vi "Csv_fill_null.vi"(8 "Data in":T1={"Initialisation"={"LMT - Connect UUT (con COM)"="Skip", "LMT - Software Version (rrel)"="Skip", "LMT - Write SKU file (wskuc)"="Skip", "LMT - SKU file name"="Skip", "Connect UUT DDM"="", "Read DDM EOL Timestamp - Mode"="", "Read DDM EOL Timestamp - Timestamp"="", "Read DDM EOL Timestamp - Rig ID"="", "Read DDM EOL Timestamp - Passmark ID"="", "Read DDM EOL Timestamp - Passmark Rev"="", "Software Version before flashing"="", "Read Hardware Serial"="", "UUT DDM SN"="", "Compare DDM SN with MES SN"="Skip", "Backup PCBA Calibration EEPROM Response - CAL"="Skip", "Flash Firmware Version"="", "Check SW Version"="", "Read DDM SW Version after flashing"="", "Set SKU Config"="", "Ready Status"="Skip", "Set Device Mode to EOL"="", "DDM Parameter - Voltage"="", "DDM Parameter - Current"="", "DDM Parameter - Power"="", "DDM Parameter - Speed"="", "DDM Parameter - Pressure"="", "Tester Parameter - Voltage"="", "Tester Parameter - Current"="", "Tester Parameter - Power"="", "Tester Parameter - Ambient Pressure"="", "Tester Parameter - Ambient Temperature"="", "Calculated Parameter - DDM Pressure Corrected"="", "Calculated Parameter - DDM Real Power"="", "Calculated Parameter - Delta V"=""}, "BEMF_Calibration"={"Calibration Result - eol_cold_bemf_temp"="", "DDM Ambient Temp"="Skip", "Restriction Plate Diameter"="Skip", "Calibration Result - eol_bemf_mp_cold_coef_a"="", "Calibration Result - eol_bemf_mp_cold_coef_b"="", "Calibration Result - eol_bemf_mp_cold_coef_c"="", "Calibration Result - eol_bemf_lsi_cold_ref_coeffs"="", "Get - Calibration Result - eol_bemf_lsi_speed"="", "Get - Calibration Result - eol_bemf_lsi_integral_0"="", "Calibration Result - eol_bemf_lsi_integral_1"="", "Get - Calibration Result - eol_bemf_lsi_integral_2"="", "Get - Calibration Result - eol_cold_bemf"="", "Get - Calibration Result - eol_cold_bemf_fisf"="", "Finalise Calibration"="Skip", "Compare -Calibration Result - eol_cold_bemf"="", "Compare -Calibration Result - eol_cold_bemf_fisf"=""}, "ECO"={"Reset Power Tune"="", "Reset BEMF FISF Calibration"="", "Restriction Plate Diameter"="", "ECO - Stabilisation Time"="", "ECO - DDM Parameter - Voltage"="", "ECO - DDM Parameter - Current"="", "ECO - DDM Parameter - Power"="", "ECO - DDM Parameter - Measured Power"="", "ECO - DDM Parameter - Speed"="", "ECO - DDM Parameter - Pressure"="", "ECO - Tester Parameter - Voltage"="", "ECO - Tester Parameter - Current"="", "ECO - Tester Parameter - Power"="", "ECO - Tester Parameter - Ambient Pressure"="", "ECO - Tester Parameter - Ambient Temperature"="", "ECO - Tester Parameter - Ambient Humidity"="", "ECO - Calculated Parameter - DDM Pressure Corrected"="", "ECO - Calculated Parameter - DDM Real Power"="", "ECO - Calculated Parameter - Delta V"="", "ECO - Calculated Parameter - Flowrate"="", "ECO - Calculated Parameter - Airwatt"="", "ECO - Formula"="", "PT ECO - Power Tune Mode Status"="Skip"}, "BOOST"={"Restriction Plate Diameter"="", "BOOST - Stabilisation Time"="", "BOOST - DDM Parameter - Voltage"="", "BOOST - DDM Parameter - Current"="", "BOOST - DDM Parameter - Power"="", "BOOST - DDM Parameter - Measured Power"="", "BOOST - DDM Parameter - Speed"="", "BOOST - DDM Parameter - Pressure"="", "BOOST - Tester Parameter - Voltage"="", "BOOST - Tester Parameter - Current"="", "BOOST - Tester Parameter - Power"="", "BOOST - Tester Parameter - Ambient Pressure"="", "BOOST - Tester Parameter - Ambient Temperature"="", "BOOST - Tester Parameter - Ambient Humidity"="", "BOOST - Calculated Parameter - DDM Pressure Corrected"="", "BOOST - Calculated Parameter - DDM Real Power"="", "BOOST - Calculated Parameter - Delta V"="", "BOOST - Calculated Parameter - Flowrate"="", "BOOST - Calculated Parameter - Airwatt"="", "BOOST - Get AM Presence"="", "Air Muscle Turn Off Status"="", "BOOST - Air Muscle Calculated Parameter - Airwatt B"="", "BOOST - Air Muscle Calculate Airwatt Delta"="", "PT BOOST - Power Tune Mode Status"="Skip", "Finalise Calibration"="Skip", "ECO - Get AW Calibration value"="", "BOOST - Get AW Calibration value"=""}, "MAX"={"Restriction Plate Diameter"="", "MAX - Stabilisation Time"="", "Get Average Delta Tmag (LSIdelta_FISFdelta_LSItmag_FISFtmag_IIRtmag)"="", "Get Average Delta Tmag FISF"="", "MAX - DDM Parameter - Voltage"="", "MAX - DDM Parameter - Current"="", "MAX - DDM Parameter - Power"="", "MAX - DDM Parameter - Measured Power"="", "MAX - DDM Parameter - Speed"="", "MAX - DDM Parameter - Pressure"="", "MAX - Tester Parameter - Voltage"="", "MAX - Tester Parameter - Current"="", "MAX - Tester Parameter - Power"="", "MAX - Tester Parameter - Ambient Pressure"="", "MAX - Tester Parameter - Ambient Temperature"="", "MAX - Tester Parameter - Ambient Humidity"="", "MAX - Calculated Parameter - DDM Pressure Corrected"="", "MAX - Calculated Parameter - DDM Real Power"="", "MAX - Calculated Parameter - Delta V"="", "MAX - Calculated Parameter - Flowrate"="", "MAX - Calculated Parameter - Airwatt"="", "MAX_FISF_Check_Average_Delta_Tmag"="", "MAX - FISF - BEMF Finetune Result"="No BEMF Finetune Required", "MAX tune - Delta P1"="No AW tune required", "MAX tune - Calculated Parameter - Airwatt"="", "Calculate Delta Airwatts - MAX finetune - Delta P2"="No AW finetune required", "MAX finetune - DDM Parameter - Voltage"="", "MAX finetune - DDM Parameter - Current"="", "MAX finetune - DDM Parameter - Power"="", "MAX finetune - DDM Parameter - Measured Power"="", "MAX finetune - DDM Parameter - Speed"="", "MAX finetune - DDM Parameter - Pressure"="", "MAX finetune - Tester Parameter - Voltage"="", "MAX finetune - Tester Parameter - Current"="", "MAX finetune - Tester Parameter - Power"="", "MAX finetune - Tester Parameter - Ambient Pressure"="", "MAX finetune - Tester Parameter - Ambient Temperature"="", "MAX finetune - Tester Parameter - Ambient Humidity"="", "MAX finetune - Calculated Parameter - DDM Pressure Corrected"="", "MAX finetune - Calculated Parameter - DDM Real Power"="", "MAX finetune - Calculated Parameter - Delta V"="", "MAX finetune - Calculated Parameter - Flowrate"="", "MAX finetune - Calculated Parameter - Airwatt"="", "Check Derate Result"="", "Delta Tmag FISF"="", "Get Hot BEMF Result"="", "Calculate delta Pressure"="", "Finalise Calibration"="Skip", "Calculate & Check Delta BEMF"="", "Delta P Airwatts Value"=""}, "LL"={"DDM Ambient Temp"="", "Restriction Plate Diameter"="", "LL - DDM Parameter - Voltage"="", "LL - DDM Parameter - Current"="", "LL - DDM Parameter - Power"="", "LL - DDM Parameter - Measured Power"="", "LL - DDM Parameter - Speed"="", "LL - DDM Parameter - Pressure"="", "LL - Tester Parameter - Voltage"="", "LL - Tester Parameter - Current"="", "LL - Tester Parameter - Power"="", "LL - DDM Real Power"="", "LL - Calibrate Task Detect LL"=""}, "HL"={"HL - DDM Parameter - Voltage"="", "HL - DDM Parameter - Current"="", "HL - DDM Parameter - Power"="", "HL - DDM Parameter - Measured Power"="", "HL - DDM Parameter - Speed"="", "HL - DDM Parameter - Pressure"="", "HL - Tester Parameter - Voltage"="", "HL - Tester Parameter - Current"="", "HL - Tester Parameter - Power"="", "HL - DDM Real Power"="", "HL - Calibrate Task Detect HL"=""}, "LH"={"Restriction Plate Diameter"="", "LH - DDM Parameter - Voltage"="", "LH - DDM Parameter - Current"="", "LH - DDM Parameter - Power"="", "LH - DDM Parameter - Measured Power"="", "LH - DDM Parameter - Speed"="", "LH - DDM Parameter - Pressure"="", "LH - Tester Parameter - Voltage"="", "LH - Tester Parameter - Current"="", "LH - Tester Parameter - Power"="", "LH - DDM Real Power"="", "LH - Calibrate Task Detect LH"=""}, "HH"={"HH - DDM Parameter - Voltage"="", "HH - DDM Parameter - Current"="", "HH - DDM Parameter - Power"="", "HH - DDM Parameter - Measured Power"="", "HH - DDM Parameter - Speed"="", "HH - DDM Parameter - Pressure"="", "HH - Tester Parameter - Voltage"="", "HH - Tester Parameter - Current"="", "HH - Tester Parameter - Power"="", "HH - DDM Real Power"="", "HH - Calibrate Task Detect HH"=""}, "Inlet Blockage Calibration"={"Inlet Blockage Calibration - DDM Parameter - Voltage"="", "Inlet Blockage Calibration - DDM Parameter - Current"="", "Inlet Blockage Calibration - DDM Parameter - Power"="", "Inlet Blockage Calibration - DDM Parameter - Measured Power"="", "Inlet Blockage Calibration - DDM Parameter - Speed"="", "Inlet Blockage Calibration - DDM Parameter - Pressure"="", "Inlet Blockage Calibration - Tester Parameter - Voltage"="", "Inlet Blockage Calibration - Tester Parameter - Current"="", "Inlet Blockage Calibration - Tester Parameter - Power"="", "Inlet Blockage Calibration - DDM Real Power"="", "Calibration Inlet Blockage_E"="", "Finalise Calibration"="Skip", "Get Task Detect LL"="", "Get Task Detect HL"="", "Get Task Detect LH"="", "Get Task Detect HH"="", "Calibration Inlet Blockage"="", "Calibration eol cold bemf temp"=""}, "GOOD"={"GOOD UNIT - Clear EEPROM Error Log"="", "GOOD UNIT - Write Product Timestamp - Mode"="", "GOOD UNIT - Write Product Timestamp - Timestamp"="", "GOOD UNIT - Write Product Timestamp - Rig ID"="", "GOOD UNIT - Write Product Timestamp - Passmark ID"="", "GOOD UNIT - Write Product Timestamp - Passmark Rev"="", "GOOD UNIT - Set Device Mode to PROD"="", "GOOD UNIT - Backup PCBA Calibration EEPROM Response"="", "GOOD UNIT - Check Security Bit"="", "GOOD UNIT - Set Calibration Lock"="", "GOOD UNIT - Get_Calibration_Lock"="", "GOOD UNIT - Disconnect UUT"=""}, "NG"={"NG UNIT - Read NVM Error"="", "NG UNIT - Set Device Mode to FCT"="", "NG UNIT - Backup PCBA Calibration EEPROM Response - CAL"="", "NG UNIT - Backup PCBA Calibration EEPROM Response - ERROR"="", "NG UNIT - Backup PCBA Calibration EEPROM Response - USAGE"="", "NG UNIT - Disconnect UUT"=""}, "SN"="", "Table"=[], "Count"={"Total"=0, "OK"=0, "NG"=0, "Yield"=0.0}, "Start Time"=timestamp(0 s since 1904-01-01), "daemon reference"=refnum, "CT"=0.0, "Config"=[], "OK/NG"=FALSE, "Station ID"="", "MES DDM SN"="Skip", "MES PCBA SN"="", "Retest"="Skip", "Lux"="", "Initialisation_Status"={"LMT - Connect UUT (con COM)"="", "LMT - Software Version (rrel)"="", "LMT - Write SKU file (wskuc)"="", "LMT - SKU file name"="", "Connect UUT DDM"="", "Read DDM EOL Timestamp - Mode"="", "Read DDM EOL Timestamp - Timestamp"="", "Read DDM EOL Timestamp - Rig ID"="", "Read DDM EOL Timestamp - Passmark ID"="", "Read DDM EOL Timestamp - Passmark Rev"="", "Software Version before flashing"="", "Read Hardware Serial"="", "UUT DDM SN"="", "Compare DDM SN with MES SN"="", "Backup PCBA Calibration EEPROM Response - CAL"="", "Flash Firmware Version"="", "Check SW Version"="", "Read DDM SW Version after flashing"="", "Set SKU Config"="", "Ready Status"="", "Set Device Mode to EOL"="", "DDM Parameter - Voltage"="", "DDM Parameter - Current"="", "DDM Parameter - Power"="", "DDM Parameter - Speed"="", "DDM Parameter - Pressure"="", "Tester Parameter - Voltage"="", "Tester Parameter - Current"="", "Tester Parameter - Power"="", "Tester Parameter - Ambient Pressure"="", "Tester Parameter - Ambient Temperature"="", "Calculated Parameter - DDM Pressure Corrected"="", "Calculated Parameter - DDM Real Power"="", "Calculated Parameter - Delta V"=""}, "BEMF_Calibration_Status"={"Calibration Result - eol_cold_bemf_temp"="", "DDM Ambient Temp"="", "Restriction Plate Diameter"="", "Calibration Result - eol_bemf_mp_cold_coef_a"="", "Calibration Result - eol_bemf_mp_cold_coef_b"="", "Calibration Result - eol_bemf_mp_cold_coef_c"="", "Calibration Result - eol_bemf_lsi_cold_ref_coeffs"="", "Get - Calibration Result - eol_bemf_lsi_speed"="", "Get - Calibration Result - eol_bemf_lsi_integral_0"="", "Calibration Result - eol_bemf_lsi_integral_1"="", "Get - Calibration Result - eol_bemf_lsi_integral_2"="", "Get - Calibration Result - eol_cold_bemf"="", "Get - Calibration Result - eol_cold_bemf_fisf"="", "Finalise Calibration"="", "Compare -Calibration Result - eol_cold_bemf"="", "Compare -Calibration Result - eol_cold_bemf_fisf"=""}, "ECO_Status"={"Reset Power Tune"="", "Reset BEMF FISF Calibration"="", "Restriction Plate Diameter"="", "ECO - Stabilisation Time"="", "ECO - DDM Parameter - Voltage"="", "ECO - DDM Parameter - Current"="", "ECO - DDM Parameter - Power"="", "ECO - DDM Parameter - Measured Power"="", "ECO - DDM Parameter - Speed"="", "ECO - DDM Parameter - Pressure"="", "ECO - Tester Parameter - Voltage"="", "ECO - Tester Parameter - Current"="", "ECO - Tester Parameter - Power"="", "ECO - Tester Parameter - Ambient Pressure"="", "ECO - Tester Parameter - Ambient Temperature"="", "ECO - Tester Parameter - Ambient Humidity"="", "ECO - Calculated Parameter - DDM Pressure Corrected"="", "ECO - Calculated Parameter - DDM Real Power"="", "ECO - Calculated Parameter - Delta V"="", "ECO - Calculated Parameter - Flowrate"="", "ECO - Calculated Parameter - Airwatt"="", "ECO - Formula"="", "PT ECO - Power Tune Mode Status"=""}, "BOOST_Status"={"Restriction Plate Diameter"="", "BOOST - Stabilisation Time"="", "BOOST - DDM Parameter - Voltage"="", "BOOST - DDM Parameter - Current"="", "BOOST - DDM Parameter - Power"="", "BOOST - DDM Parameter - Measured Power"="", "BOOST - DDM Parameter - Speed"="", "BOOST - DDM Parameter - Pressure"="", "BOOST - Tester Parameter - Voltage"="", "BOOST - Tester Parameter - Current"="", "BOOST - Tester Parameter - Power"="", "BOOST - Tester Parameter - Ambient Pressure"="", "BOOST - Tester Parameter - Ambient Temperature"="", "BOOST - Tester Parameter - Ambient Humidity"="", "BOOST - Calculated Parameter - DDM Pressure Corrected"="", "BOOST - Calculated Parameter - DDM Real Power"="", "BOOST - Calculated Parameter - Delta V"="", "BOOST - Calculated Parameter - Flowrate"="", "BOOST - Calculated Parameter - Airwatt"="", "BOOST - Get AM Presence"="", "Air Muscle Turn Off Status"="", "BOOST - Air Muscle Calculated Parameter - Airwatt B"="", "BOOST - Air Muscle Calculate Airwatt Delta"="", "PT BOOST - Power Tune Mode Status"="", "Finalise Calibration"="", "ECO - Get AW Calibration value"="", "BOOST - Get AW Calibration value"=""}, "MAX_Status"={"Restriction Plate Diameter"="", "MAX - Stabilisation Time"="", "Get Average Delta Tmag (LSIdelta_FISFdelta_LSItmag_FISFtmag_IIRtmag)"="", "Get Average Delta Tmag FISF"="", "MAX - DDM Parameter - Voltage"="", "MAX - DDM Parameter - Current"="", "MAX - DDM Parameter - Power"="", "MAX - DDM Parameter - Measured Power"="", "MAX - DDM Parameter - Speed"="", "MAX - DDM Parameter - Pressure"="", "MAX - Tester Parameter - Voltage"="", "MAX - Tester Parameter - Current"="", "MAX - Tester Parameter - Power"="", "MAX - Tester Parameter - Ambient Pressure"="", "MAX - Tester Parameter - Ambient Temperature"="", "MAX - Tester Parameter - Ambient Humidity"="", "MAX - Calculated Parameter - DDM Pressure Corrected"="", "MAX - Calculated Parameter - DDM Real Power"="", "MAX - Calculated Parameter - Delta V"="", "MAX - Calculated Parameter - Flowrate"="", "MAX - Calculated Parameter - Airwatt"="", "MAX_FISF_Check_Average_Delta_Tmag"="", "MAX - FISF - BEMF Finetune Result"="", "MAX tune - Delta P1"="", "MAX tune - Calculated Parameter - Airwatt"="", "Calculate Delta Airwatts - MAX finetune - Delta P2"="", "MAX finetune - DDM Parameter - Voltage"="", "MAX finetune - DDM Parameter - Current"="", "MAX finetune - DDM Parameter - Power"="", "MAX finetune - DDM Parameter - Measured Power"="", "MAX finetune - DDM Parameter - Speed"="", "MAX finetune - DDM Parameter - Pressure"="", "MAX finetune - Tester Parameter - Voltage"="", "MAX finetune - Tester Parameter - Current"="", "MAX finetune - Tester Parameter - Power"="", "MAX finetune - Tester Parameter - Ambient Pressure"="", "MAX finetune - Tester Parameter - Ambient Temperature"="", "MAX finetune - Tester Parameter - Ambient Humidity"="", "MAX finetune - Calculated Parameter - DDM Pressure Corrected"="", "MAX finetune - Calculated Parameter - DDM Real Power"="", "MAX finetune - Calculated Parameter - Delta V"="", "MAX finetune - Calculated Parameter - Flowrate"="", "MAX finetune - Calculated Parameter - Airwatt"="", "Check Derate Result"="", "Delta Tmag FISF"="", "Get Hot BEMF Result"="", "Calculate delta Pressure"="", "Finalise Calibration"="", "Calculate & Check Delta BEMF"="", "Delta P Airwatts Value"=""}, "LL_Status"={"DDM Ambient Temp"="", "Restriction Plate Diameter"="", "LL - DDM Parameter - Voltage"="", "LL - DDM Parameter - Current"="", "LL - DDM Parameter - Power"="", "LL - DDM Parameter - Measured Power"="", "LL - DDM Parameter - Speed"="", "LL - DDM Parameter - Pressure"="", "LL - Tester Parameter - Voltage"="", "LL - Tester Parameter - Current"="", "LL - Tester Parameter - Power"="", "LL - DDM Real Power"="", "LL - Calibrate Task Detect LL"=""}, "HL_Status"={"HL - DDM Parameter - Voltage"="", "HL - DDM Parameter - Current"="", "HL - DDM Parameter - Power"="", "HL - DDM Parameter - Measured Power"="", "HL - DDM Parameter - Speed"="", "HL - DDM Parameter - Pressure"="", "HL - Tester Parameter - Voltage"="", "HL - Tester Parameter - Current"="", "HL - Tester Parameter - Power"="", "HL - DDM Real Power"="", "HL - Calibrate Task Detect HL"=""}, "LH_Status"={"Restriction Plate Diameter"="", "LH - DDM Parameter - Voltage"="", "LH - DDM Parameter - Current"="", "LH - DDM Parameter - Power"="", "LH - DDM Parameter - Measured Power"="", "LH - DDM Parameter - Speed"="", "LH - DDM Parameter - Pressure"="", "LH - Tester Parameter - Voltage"="", "LH - Tester Parameter - Current"="", "LH - Tester Parameter - Power"="", "LH - DDM Real Power"="", "LH - Calibrate Task Detect LH"=""}, "HH_Status"={"HH - DDM Parameter - Voltage"="", "HH - DDM Parameter - Current"="", "HH - DDM Parameter - Power"="", "HH - DDM Parameter - Measured Power"="", "HH - DDM Parameter - Speed"="", "HH - DDM Parameter - Pressure"="", "HH - Tester Parameter - Voltage"="", "HH - Tester Parameter - Current"="", "HH - Tester Parameter - Power"="", "HH - DDM Real Power"="", "HH - Calibrate Task Detect HH"=""}, "Inlet Blockage Calibration_Status"={"Inlet Blockage Calibration - DDM Parameter - Voltage"="", "Inlet Blockage Calibration - DDM Parameter - Current"="", "Inlet Blockage Calibration - DDM Parameter - Power"="", "Inlet Blockage Calibration - DDM Parameter - Measured Power"="", "Inlet Blockage Calibration - DDM Parameter - Speed"="", "Inlet Blockage Calibration - DDM Parameter - Pressure"="", "Inlet Blockage Calibration - Tester Parameter - Voltage"="", "Inlet Blockage Calibration - Tester Parameter - Current"="", "Inlet Blockage Calibration - Tester Parameter - Power"="", "Inlet Blockage Calibration - DDM Real Power"="", "Calibration Inlet Blockage_E"="", "Finalise Calibration"="", "Get Task Detect LL"="", "Get Task Detect HL"="", "Get Task Detect LH"="", "Get Task Detect HH"="", "Calibration Inlet Blockage"="", "Calibration eol cold bemf temp"=""}, "GOOD_Status"={"GOOD UNIT - Clear EEPROM Error Log"="", "GOOD UNIT - Write Product Timestamp - Mode"="", "GOOD UNIT - Write Product Timestamp - Timestamp"="", "GOOD UNIT - Write Product Timestamp - Rig ID"="", "GOOD UNIT - Write Product Timestamp - Passmark ID"="", "GOOD UNIT - Write Product Timestamp - Passmark Rev"="", "GOOD UNIT - Set Device Mode to PROD"="", "GOOD UNIT - Backup PCBA Calibration EEPROM Response"="", "GOOD UNIT - Check Security Bit"="", "GOOD UNIT - Set Calibration Lock"="", "GOOD UNIT - Get_Calibration_Lock"="", "GOOD UNIT - Disconnect UUT"=""}, "NG_Status"={"NG UNIT - Read NVM Error"="", "NG UNIT - Set Device Mode to FCT"="", "NG UNIT - Backup PCBA Calibration EEPROM Response - CAL"="", "NG UNIT - Backup PCBA Calibration EEPROM Response - ERROR"="", "NG UNIT - Backup PCBA Calibration EEPROM Response - USAGE"="", "NG UNIT - Disconnect UUT"=""}, "SKU"="", "Plate_Diameter"="", "Alarm"=""}) -> (0 "Data out":T1={"Initialisation"={"LMT - Connect UUT (con COM)"="Skip", "LMT - Software Version (rrel)"="Skip", "LMT - Write SKU file (wskuc)"="Skip", "LMT - SKU file name"="Skip", "Connect UUT DDM"="", "Read DDM EOL Timestamp - Mode"="", "Read DDM EOL Timestamp - Timestamp"="", "Read DDM EOL Timestamp - Rig ID"="", "Read DDM EOL Timestamp - Passmark ID"="", "Read DDM EOL Timestamp - Passmark Rev"="", "Software Version before flashing"="", "Read Hardware Serial"="", "UUT DDM SN"="", "Compare DDM SN with MES SN"="Skip", "Backup PCBA Calibration EEPROM Response - CAL"="Skip", "Flash Firmware Version"="", "Check SW Version"="", "Read DDM SW Version after flashing"="", "Set SKU Config"="", "Ready Status"="Skip", "Set Device Mode to EOL"="", "DDM Parameter - Voltage"="", "DDM Parameter - Current"="", "DDM Parameter - Power"="", "DDM Parameter - Speed"="", "DDM Parameter - Pressure"="", "Tester Parameter - Voltage"="", "Tester Parameter - Current"="", "Tester Parameter - Power"="", "Tester Parameter - Ambient Pressure"="", "Tester Parameter - Ambient Temperature"="", "Calculated Parameter - DDM Pressure Corrected"="", "Calculated Parameter - DDM Real Power"="", "Calculated Parameter - Delta V"=""}, "BEMF_Calibration"={"Calibration Result - eol_cold_bemf_temp"="", "DDM Ambient Temp"="Skip", "Restriction Plate Diameter"="Skip", "Calibration Result - eol_bemf_mp_cold_coef_a"="", "Calibration Result - eol_bemf_mp_cold_coef_b"="", "Calibration Result - eol_bemf_mp_cold_coef_c"="", "Calibration Result - eol_bemf_lsi_cold_ref_coeffs"="", "Get - Calibration Result - eol_bemf_lsi_speed"="", "Get - Calibration Result - eol_bemf_lsi_integral_0"="", "Calibration Result - eol_bemf_lsi_integral_1"="", "Get - Calibration Result - eol_bemf_lsi_integral_2"="", "Get - Calibration Result - eol_cold_bemf"="", "Get - Calibration Result - eol_cold_bemf_fisf"="", "Finalise Calibration"="Skip", "Compare -Calibration Result - eol_cold_bemf"="", "Compare -Calibration Result - eol_cold_bemf_fisf"=""}, "ECO"={"Reset Power Tune"="", "Reset BEMF FISF Calibration"="", "Restriction Plate Diameter"="", "ECO - Stabilisation Time"="", "ECO - DDM Parameter - Voltage"="", "ECO - DDM Parameter - Current"="", "ECO - DDM Parameter - Power"="", "ECO - DDM Parameter - Measured Power"="", "ECO - DDM Parameter - Speed"="", "ECO - DDM Parameter - Pressure"="", "ECO - Tester Parameter - Voltage"="", "ECO - Tester Parameter - Current"="", "ECO - Tester Parameter - Power"="", "ECO - Tester Parameter - Ambient Pressure"="", "ECO - Tester Parameter - Ambient Temperature"="", "ECO - Tester Parameter - Ambient Humidity"="", "ECO - Calculated Parameter - DDM Pressure Corrected"="", "ECO - Calculated Parameter - DDM Real Power"="", "ECO - Calculated Parameter - Delta V"="", "ECO - Calculated Parameter - Flowrate"="", "ECO - Calculated Parameter - Airwatt"="", "ECO - Formula"="", "PT ECO - Power Tune Mode Status"="Skip"}, "BOOST"={"Restriction Plate Diameter"="", "BOOST - Stabilisation Time"="", "BOOST - DDM Parameter - Voltage"="", "BOOST - DDM Parameter - Current"="", "BOOST - DDM Parameter - Power"="", "BOOST - DDM Parameter - Measured Power"="", "BOOST - DDM Parameter - Speed"="", "BOOST - DDM Parameter - Pressure"="", "BOOST - Tester Parameter - Voltage"="", "BOOST - Tester Parameter - Current"="", "BOOST - Tester Parameter - Power"="", "BOOST - Tester Parameter - Ambient Pressure"="", "BOOST - Tester Parameter - Ambient Temperature"="", "BOOST - Tester Parameter - Ambient Humidity"="", "BOOST - Calculated Parameter - DDM Pressure Corrected"="", "BOOST - Calculated Parameter - DDM Real Power"="", "BOOST - Calculated Parameter - Delta V"="", "BOOST - Calculated Parameter - Flowrate"="", "BOOST - Calculated Parameter - Airwatt"="", "BOOST - Get AM Presence"="", "Air Muscle Turn Off Status"="", "BOOST - Air Muscle Calculated Parameter - Airwatt B"="", "BOOST - Air Muscle Calculate Airwatt Delta"="", "PT BOOST - Power Tune Mode Status"="Skip", "Finalise Calibration"="Skip", "ECO - Get AW Calibration value"="", "BOOST - Get AW Calibration value"=""}, "MAX"={"Restriction Plate Diameter"="", "MAX - Stabilisation Time"="", "Get Average Delta Tmag (LSIdelta_FISFdelta_LSItmag_FISFtmag_IIRtmag)"="", "Get Average Delta Tmag FISF"="", "MAX - DDM Parameter - Voltage"="", "MAX - DDM Parameter - Current"="", "MAX - DDM Parameter - Power"="", "MAX - DDM Parameter - Measured Power"="", "MAX - DDM Parameter - Speed"="", "MAX - DDM Parameter - Pressure"="", "MAX - Tester Parameter - Voltage"="", "MAX - Tester Parameter - Current"="", "MAX - Tester Parameter - Power"="", "MAX - Tester Parameter - Ambient Pressure"="", "MAX - Tester Parameter - Ambient Temperature"="", "MAX - Tester Parameter - Ambient Humidity"="", "MAX - Calculated Parameter - DDM Pressure Corrected"="", "MAX - Calculated Parameter - DDM Real Power"="", "MAX - Calculated Parameter - Delta V"="", "MAX - Calculated Parameter - Flowrate"="", "MAX - Calculated Parameter - Airwatt"="", "MAX_FISF_Check_Average_Delta_Tmag"="", "MAX - FISF - BEMF Finetune Result"="No BEMF Finetune Required", "MAX tune - Delta P1"="No AW tune required", "MAX tune - Calculated Parameter - Airwatt"="", "Calculate Delta Airwatts - MAX finetune - Delta P2"="No AW finetune required", "MAX finetune - DDM Parameter - Voltage"="", "MAX finetune - DDM Parameter - Current"="", "MAX finetune - DDM Parameter - Power"="", "MAX finetune - DDM Parameter - Measured Power"="", "MAX finetune - DDM Parameter - Speed"="", "MAX finetune - DDM Parameter - Pressure"="", "MAX finetune - Tester Parameter - Voltage"="", "MAX finetune - Tester Parameter - Current"="", "MAX finetune - Tester Parameter - Power"="", "MAX finetune - Tester Parameter - Ambient Pressure"="", "MAX finetune - Tester Parameter - Ambient Temperature"="", "MAX finetune - Tester Parameter - Ambient Humidity"="", "MAX finetune - Calculated Parameter - DDM Pressure Corrected"="", "MAX finetune - Calculated Parameter - DDM Real Power"="", "MAX finetune - Calculated Parameter - Delta V"="", "MAX finetune - Calculated Parameter - Flowrate"="", "MAX finetune - Calculated Parameter - Airwatt"="", "Check Derate Result"="", "Delta Tmag FISF"="", "Get Hot BEMF Result"="", "Calculate delta Pressure"="", "Finalise Calibration"="Skip", "Calculate & Check Delta BEMF"="", "Delta P Airwatts Value"=""}, "LL"={"DDM Ambient Temp"="", "Restriction Plate Diameter"="", "LL - DDM Parameter - Voltage"="", "LL - DDM Parameter - Current"="", "LL - DDM Parameter - Power"="", "LL - DDM Parameter - Measured Power"="", "LL - DDM Parameter - Speed"="", "LL - DDM Parameter - Pressure"="", "LL - Tester Parameter - Voltage"="", "LL - Tester Parameter - Current"="", "LL - Tester Parameter - Power"="", "LL - DDM Real Power"="", "LL - Calibrate Task Detect LL"=""}, "HL"={"HL - DDM Parameter - Voltage"="", "HL - DDM Parameter - Current"="", "HL - DDM Parameter - Power"="", "HL - DDM Parameter - Measured Power"="", "HL - DDM Parameter - Speed"="", "HL - DDM Parameter - Pressure"="", "HL - Tester Parameter - Voltage"="", "HL - Tester Parameter - Current"="", "HL - Tester Parameter - Power"="", "HL - DDM Real Power"="", "HL - Calibrate Task Detect HL"=""}, "LH"={"Restriction Plate Diameter"="", "LH - DDM Parameter - Voltage"="", "LH - DDM Parameter - Current"="", "LH - DDM Parameter - Power"="", "LH - DDM Parameter - Measured Power"="", "LH - DDM Parameter - Speed"="", "LH - DDM Parameter - Pressure"="", "LH - Tester Parameter - Voltage"="", "LH - Tester Parameter - Current"="", "LH - Tester Parameter - Power"="", "LH - DDM Real Power"="", "LH - Calibrate Task Detect LH"=""}, "HH"={"HH - DDM Parameter - Voltage"="", "HH - DDM Parameter - Current"="", "HH - DDM Parameter - Power"="", "HH - DDM Parameter - Measured Power"="", "HH - DDM Parameter - Speed"="", "HH - DDM Parameter - Pressure"="", "HH - Tester Parameter - Voltage"="", "HH - Tester Parameter - Current"="", "HH - Tester Parameter - Power"="", "HH - DDM Real Power"="", "HH - Calibrate Task Detect HH"=""}, "Inlet Blockage Calibration"={"Inlet Blockage Calibration - DDM Parameter - Voltage"="", "Inlet Blockage Calibration - DDM Parameter - Current"="", "Inlet Blockage Calibration - DDM Parameter - Power"="", "Inlet Blockage Calibration - DDM Parameter - Measured Power"="", "Inlet Blockage Calibration - DDM Parameter - Speed"="", "Inlet Blockage Calibration - DDM Parameter - Pressure"="", "Inlet Blockage Calibration - Tester Parameter - Voltage"="", "Inlet Blockage Calibration - Tester Parameter - Current"="", "Inlet Blockage Calibration - Tester Parameter - Power"="", "Inlet Blockage Calibration - DDM Real Power"="", "Calibration Inlet Blockage_E"="", "Finalise Calibration"="Skip", "Get Task Detect LL"="", "Get Task Detect HL"="", "Get Task Detect LH"="", "Get Task Detect HH"="", "Calibration Inlet Blockage"="", "Calibration eol cold bemf temp"=""}, "GOOD"={"GOOD UNIT - Clear EEPROM Error Log"="", "GOOD UNIT - Write Product Timestamp - Mode"="", "GOOD UNIT - Write Product Timestamp - Timestamp"="", "GOOD UNIT - Write Product Timestamp - Rig ID"="", "GOOD UNIT - Write Product Timestamp - Passmark ID"="", "GOOD UNIT - Write Product Timestamp - Passmark Rev"="", "GOOD UNIT - Set Device Mode to PROD"="", "GOOD UNIT - Backup PCBA Calibration EEPROM Response"="", "GOOD UNIT - Check Security Bit"="", "GOOD UNIT - Set Calibration Lock"="", "GOOD UNIT - Get_Calibration_Lock"="", "GOOD UNIT - Disconnect UUT"=""}, "NG"={"NG UNIT - Read NVM Error"="", "NG UNIT - Set Device Mode to FCT"="", "NG UNIT - Backup PCBA Calibration EEPROM Response - CAL"="", "NG UNIT - Backup PCBA Calibration EEPROM Response - ERROR"="", "NG UNIT - Backup PCBA Calibration EEPROM Response - USAGE"="", "NG UNIT - Disconnect UUT"=""}, "SN"="", "Table"=[], "Count"={"Total"=0, "OK"=0, "NG"=0, "Yield"=0.0}, "Start Time"=timestamp(0 s since 1904-01-01), "daemon reference"=refnum, "CT"=0.0, "Config"=[], "OK/NG"=FALSE, "Station ID"="", "MES DDM SN"="Skip", "MES PCBA SN"="", "Retest"="Skip", "Lux"="", "Initialisation_Status"={"LMT - Connect UUT (con COM)"="", "LMT - Software Version (rrel)"="", "LMT - Write SKU file (wskuc)"="", "LMT - SKU file name"="", "Connect UUT DDM"="", "Read DDM EOL Timestamp - Mode"="", "Read DDM EOL Timestamp - Timestamp"="", "Read DDM EOL Timestamp - Rig ID"="", "Read DDM EOL Timestamp - Passmark ID"="", "Read DDM EOL Timestamp - Passmark Rev"="", "Software Version before flashing"="", "Read Hardware Serial"="", "UUT DDM SN"="", "Compare DDM SN with MES SN"="", "Backup PCBA Calibration EEPROM Response - CAL"="", "Flash Firmware Version"="", "Check SW Version"="", "Read DDM SW Version after flashing"="", "Set SKU Config"="", "Ready Status"="", "Set Device Mode to EOL"="", "DDM Parameter - Voltage"="", "DDM Parameter - Current"="", "DDM Parameter - Power"="", "DDM Parameter - Speed"="", "DDM Parameter - Pressure"="", "Tester Parameter - Voltage"="", "Tester Parameter - Current"="", "Tester Parameter - Power"="", "Tester Parameter - Ambient Pressure"="", "Tester Parameter - Ambient Temperature"="", "Calculated Parameter - DDM Pressure Corrected"="", "Calculated Parameter - DDM Real Power"="", "Calculated Parameter - Delta V"=""}, "BEMF_Calibration_Status"={"Calibration Result - eol_cold_bemf_temp"="", "DDM Ambient Temp"="", "Restriction Plate Diameter"="", "Calibration Result - eol_bemf_mp_cold_coef_a"="", "Calibration Result - eol_bemf_mp_cold_coef_b"="", "Calibration Result - eol_bemf_mp_cold_coef_c"="", "Calibration Result - eol_bemf_lsi_cold_ref_coeffs"="", "Get - Calibration Result - eol_bemf_lsi_speed"="", "Get - Calibration Result - eol_bemf_lsi_integral_0"="", "Calibration Result - eol_bemf_lsi_integral_1"="", "Get - Calibration Result - eol_bemf_lsi_integral_2"="", "Get - Calibration Result - eol_cold_bemf"="", "Get - Calibration Result - eol_cold_bemf_fisf"="", "Finalise Calibration"="", "Compare -Calibration Result - eol_cold_bemf"="", "Compare -Calibration Result - eol_cold_bemf_fisf"=""}, "ECO_Status"={"Reset Power Tune"="", "Reset BEMF FISF Calibration"="", "Restriction Plate Diameter"="", "ECO - Stabilisation Time"="", "ECO - DDM Parameter - Voltage"="", "ECO - DDM Parameter - Current"="", "ECO - DDM Parameter - Power"="", "ECO - DDM Parameter - Measured Power"="", "ECO - DDM Parameter - Speed"="", "ECO - DDM Parameter - Pressure"="", "ECO - Tester Parameter - Voltage"="", "ECO - Tester Parameter - Current"="", "ECO - Tester Parameter - Power"="", "ECO - Tester Parameter - Ambient Pressure"="", "ECO - Tester Parameter - Ambient Temperature"="", "ECO - Tester Parameter - Ambient Humidity"="", "ECO - Calculated Parameter - DDM Pressure Corrected"="", "ECO - Calculated Parameter - DDM Real Power"="", "ECO - Calculated Parameter - Delta V"="", "ECO - Calculated Parameter - Flowrate"="", "ECO - Calculated Parameter - Airwatt"="", "ECO - Formula"="", "PT ECO - Power Tune Mode Status"=""}, "BOOST_Status"={"Restriction Plate Diameter"="", "BOOST - Stabilisation Time"="", "BOOST - DDM Parameter - Voltage"="", "BOOST - DDM Parameter - Current"="", "BOOST - DDM Parameter - Power"="", "BOOST - DDM Parameter - Measured Power"="", "BOOST - DDM Parameter - Speed"="", "BOOST - DDM Parameter - Pressure"="", "BOOST - Tester Parameter - Voltage"="", "BOOST - Tester Parameter - Current"="", "BOOST - Tester Parameter - Power"="", "BOOST - Tester Parameter - Ambient Pressure"="", "BOOST - Tester Parameter - Ambient Temperature"="", "BOOST - Tester Parameter - Ambient Humidity"="", "BOOST - Calculated Parameter - DDM Pressure Corrected"="", "BOOST - Calculated Parameter - DDM Real Power"="", "BOOST - Calculated Parameter - Delta V"="", "BOOST - Calculated Parameter - Flowrate"="", "BOOST - Calculated Parameter - Airwatt"="", "BOOST - Get AM Presence"="", "Air Muscle Turn Off Status"="", "BOOST - Air Muscle Calculated Parameter - Airwatt B"="", "BOOST - Air Muscle Calculate Airwatt Delta"="", "PT BOOST - Power Tune Mode Status"="", "Finalise Calibration"="", "ECO - Get AW Calibration value"="", "BOOST - Get AW Calibration value"=""}, "MAX_Status"={"Restriction Plate Diameter"="", "MAX - Stabilisation Time"="", "Get Average Delta Tmag (LSIdelta_FISFdelta_LSItmag_FISFtmag_IIRtmag)"="", "Get Average Delta Tmag FISF"="", "MAX - DDM Parameter - Voltage"="", "MAX - DDM Parameter - Current"="", "MAX - DDM Parameter - Power"="", "MAX - DDM Parameter - Measured Power"="", "MAX - DDM Parameter - Speed"="", "MAX - DDM Parameter - Pressure"="", "MAX - Tester Parameter - Voltage"="", "MAX - Tester Parameter - Current"="", "MAX - Tester Parameter - Power"="", "MAX - Tester Parameter - Ambient Pressure"="", "MAX - Tester Parameter - Ambient Temperature"="", "MAX - Tester Parameter - Ambient Humidity"="", "MAX - Calculated Parameter - DDM Pressure Corrected"="", "MAX - Calculated Parameter - DDM Real Power"="", "MAX - Calculated Parameter - Delta V"="", "MAX - Calculated Parameter - Flowrate"="", "MAX - Calculated Parameter - Airwatt"="", "MAX_FISF_Check_Average_Delta_Tmag"="", "MAX - FISF - BEMF Finetune Result"="", "MAX tune - Delta P1"="", "MAX tune - Calculated Parameter - Airwatt"="", "Calculate Delta Airwatts - MAX finetune - Delta P2"="", "MAX finetune - DDM Parameter - Voltage"="", "MAX finetune - DDM Parameter - Current"="", "MAX finetune - DDM Parameter - Power"="", "MAX finetune - DDM Parameter - Measured Power"="", "MAX finetune - DDM Parameter - Speed"="", "MAX finetune - DDM Parameter - Pressure"="", "MAX finetune - Tester Parameter - Voltage"="", "MAX finetune - Tester Parameter - Current"="", "MAX finetune - Tester Parameter - Power"="", "MAX finetune - Tester Parameter - Ambient Pressure"="", "MAX finetune - Tester Parameter - Ambient Temperature"="", "MAX finetune - Tester Parameter - Ambient Humidity"="", "MAX finetune - Calculated Parameter - DDM Pressure Corrected"="", "MAX finetune - Calculated Parameter - DDM Real Power"="", "MAX finetune - Calculated Parameter - Delta V"="", "MAX finetune - Calculated Parameter - Flowrate"="", "MAX finetune - Calculated Parameter - Airwatt"="", "Check Derate Result"="", "Delta Tmag FISF"="", "Get Hot BEMF Result"="", "Calculate delta Pressure"="", "Finalise Calibration"="", "Calculate & Check Delta BEMF"="", "Delta P Airwatts Value"=""}, "LL_Status"={"DDM Ambient Temp"="", "Restriction Plate Diameter"="", "LL - DDM Parameter - Voltage"="", "LL - DDM Parameter - Current"="", "LL - DDM Parameter - Power"="", "LL - DDM Parameter - Measured Power"="", "LL - DDM Parameter - Speed"="", "LL - DDM Parameter - Pressure"="", "LL - Tester Parameter - Voltage"="", "LL - Tester Parameter - Current"="", "LL - Tester Parameter - Power"="", "LL - DDM Real Power"="", "LL - Calibrate Task Detect LL"=""}, "HL_Status"={"HL - DDM Parameter - Voltage"="", "HL - DDM Parameter - Current"="", "HL - DDM Parameter - Power"="", "HL - DDM Parameter - Measured Power"="", "HL - DDM Parameter - Speed"="", "HL - DDM Parameter - Pressure"="", "HL - Tester Parameter - Voltage"="", "HL - Tester Parameter - Current"="", "HL - Tester Parameter - Power"="", "HL - DDM Real Power"="", "HL - Calibrate Task Detect HL"=""}, "LH_Status"={"Restriction Plate Diameter"="", "LH - DDM Parameter - Voltage"="", "LH - DDM Parameter - Current"="", "LH - DDM Parameter - Power"="", "LH - DDM Parameter - Measured Power"="", "LH - DDM Parameter - Speed"="", "LH - DDM Parameter - Pressure"="", "LH - Tester Parameter - Voltage"="", "LH - Tester Parameter - Current"="", "LH - Tester Parameter - Power"="", "LH - DDM Real Power"="", "LH - Calibrate Task Detect LH"=""}, "HH_Status"={"HH - DDM Parameter - Voltage"="", "HH - DDM Parameter - Current"="", "HH - DDM Parameter - Power"="", "HH - DDM Parameter - Measured Power"="", "HH - DDM Parameter - Speed"="", "HH - DDM Parameter - Pressure"="", "HH - Tester Parameter - Voltage"="", "HH - Tester Parameter - Current"="", "HH - Tester Parameter - Power"="", "HH - DDM Real Power"="", "HH - Calibrate Task Detect HH"=""}, "Inlet Blockage Calibration_Status"={"Inlet Blockage Calibration - DDM Parameter - Voltage"="", "Inlet Blockage Calibration - DDM Parameter - Current"="", "Inlet Blockage Calibration - DDM Parameter - Power"="", "Inlet Blockage Calibration - DDM Parameter - Measured Power"="", "Inlet Blockage Calibration - DDM Parameter - Speed"="", "Inlet Blockage Calibration - DDM Parameter - Pressure"="", "Inlet Blockage Calibration - Tester Parameter - Voltage"="", "Inlet Blockage Calibration - Tester Parameter - Current"="", "Inlet Blockage Calibration - Tester Parameter - Power"="", "Inlet Blockage Calibration - DDM Real Power"="", "Calibration Inlet Blockage_E"="", "Finalise Calibration"="", "Get Task Detect LL"="", "Get Task Detect HL"="", "Get Task Detect LH"="", "Get Task Detect HH"="", "Calibration Inlet Blockage"="", "Calibration eol cold bemf temp"=""}, "GOOD_Status"={"GOOD UNIT - Clear EEPROM Error Log"="", "GOOD UNIT - Write Product Timestamp - Mode"="", "GOOD UNIT - Write Product Timestamp - Timestamp"="", "GOOD UNIT - Write Product Timestamp - Rig ID"="", "GOOD UNIT - Write Product Timestamp - Passmark ID"="", "GOOD UNIT - Write Product Timestamp - Passmark Rev"="", "GOOD UNIT - Set Device Mode to PROD"="", "GOOD UNIT - Backup PCBA Calibration EEPROM Response"="", "GOOD UNIT - Check Security Bit"="", "GOOD UNIT - Set Calibration Lock"="", "GOOD UNIT - Get_Calibration_Lock"="", "GOOD UNIT - Disconnect UUT"=""}, "NG_Status"={"NG UNIT - Read NVM Error"="", "NG UNIT - Set Device Mode to FCT"="", "NG UNIT - Backup PCBA Calibration EEPROM Response - CAL"="", "NG UNIT - Backup PCBA Calibration EEPROM Response - ERROR"="", "NG UNIT - Backup PCBA Calibration EEPROM Response - USAGE"="", "NG UNIT - Disconnect UUT"=""}, "SKU"="", "Plate_Diameter"="", "Alarm"=""})   [LabVIEW 2017]
uses:
  Ctrls/CSV_Data.ctl
types:
  T1 = typedef "CSV_Data.ctl" = cluster{"Initialisation":cluster{"LMT - Connect UUT (con COM)":string, "LMT - Software Version (rrel)":string, "LMT - Write SKU file (wskuc)":string, "LMT - SKU file name":string, "Connect UUT DDM":string, "Read DDM EOL Timestamp - Mode":string, "Read DDM EOL Timestamp - Timestamp":string, "Read DDM EOL Timestamp - Rig ID":string, "Read DDM EOL Timestamp - Passmark ID":string, "Read DDM EOL Timestamp - Passmark Rev":string, "Software Version before flashing":string, "Read Hardware Serial":string, "UUT DDM SN":string, "Compare DDM SN with MES SN":string, "Backup PCBA Calibration EEPROM Response - CAL":string, "Flash Firmware Version":string, "Check SW Version":string, "Read DDM SW Version after flashing":string, "Set SKU Config":string, "Ready Status":string, "Set Device Mode to EOL":string, "DDM Parameter - Voltage":string, "DDM Parameter - Current":string, "DDM Parameter - Power":string, "DDM Parameter - Speed":string, "DDM Parameter - Pressure":string, "Tester Parameter - Voltage":string, "Tester Parameter - Current":string, "Tester Parameter - Power":string, "Tester Parameter - Ambient Pressure":string, "Tester Parameter - Ambient Temperature":string, "Calculated Parameter - DDM Pressure Corrected":string, "Calculated Parameter - DDM Real Power":string, "Calculated Parameter - Delta V":string}, "BEMF_Calibration":cluster{"Calibration Result - eol_cold_bemf_temp":string, "DDM Ambient Temp":string, "Restriction Plate Diameter":string, "Calibration Result - eol_bemf_mp_cold_coef_a":string, "Calibration Result - eol_bemf_mp_cold_coef_b":string, "Calibration Result - eol_bemf_mp_cold_coef_c":string, "Calibration Result - eol_bemf_lsi_cold_ref_coeffs":string, "Get - Calibration Result - eol_bemf_lsi_speed":string, "Get - Calibration Result - eol_bemf_lsi_integral_0":string, "Calibration Result - eol_bemf_lsi_integral_1":string, "Get - Calibration Result - eol_bemf_lsi_integral_2":string, "Get - Calibration Result - eol_cold_bemf":string, "Get - Calibration Result - eol_cold_bemf_fisf":string, "Finalise Calibration":string, "Compare -Calibration Result - eol_cold_bemf":string, "Compare -Calibration Result - eol_cold_bemf_fisf":string}, "ECO":cluster{"Reset Power Tune":string, "Reset BEMF FISF Calibration":string, "Restriction Plate Diameter":string, "ECO - Stabilisation Time":string, "ECO - DDM Parameter - Voltage":string, "ECO - DDM Parameter - Current":string, "ECO - DDM Parameter - Power":string, "ECO - DDM Parameter - Measured Power":string, "ECO - DDM Parameter - Speed":string, "ECO - DDM Parameter - Pressure":string, "ECO - Tester Parameter - Voltage":string, "ECO - Tester Parameter - Current":string, "ECO - Tester Parameter - Power":string, "ECO - Tester Parameter - Ambient Pressure":string, "ECO - Tester Parameter - Ambient Temperature":string, "ECO - Tester Parameter - Ambient Humidity":string, "ECO - Calculated Parameter - DDM Pressure Corrected":string, "ECO - Calculated Parameter - DDM Real Power":string, "ECO - Calculated Parameter - Delta V":string, "ECO - Calculated Parameter - Flowrate":string, "ECO - Calculated Parameter - Airwatt":string, "ECO - Formula":string, "PT ECO - Power Tune Mode Status":string}, "BOOST":cluster{"Restriction Plate Diameter":string, "BOOST - Stabilisation Time":string, "BOOST - DDM Parameter - Voltage":string, "BOOST - DDM Parameter - Current":string, "BOOST - DDM Parameter - Power":string, "BOOST - DDM Parameter - Measured Power":string, "BOOST - DDM Parameter - Speed":string, "BOOST - DDM Parameter - Pressure":string, "BOOST - Tester Parameter - Voltage":string, "BOOST - Tester Parameter - Current":string, "BOOST - Tester Parameter - Power":string, "BOOST - Tester Parameter - Ambient Pressure":string, "BOOST - Tester Parameter - Ambient Temperature":string, "BOOST - Tester Parameter - Ambient Humidity":string, "BOOST - Calculated Parameter - DDM Pressure Corrected":string, "BOOST - Calculated Parameter - DDM Real Power":string, "BOOST - Calculated Parameter - Delta V":string, "BOOST - Calculated Parameter - Flowrate":string, "BOOST - Calculated Parameter - Airwatt":string, "BOOST - Get AM Presence":string, "Air Muscle Turn Off Status":string, "BOOST - Air Muscle Calculated Parameter - Airwatt B":string, "BOOST - Air Muscle Calculate Airwatt Delta":string, "PT BOOST - Power Tune Mode Status":string, "Finalise Calibration":string, "ECO - Get AW Calibration value":string, "BOOST - Get AW Calibration value":string}, "MAX":cluster{"Restriction Plate Diameter":string, "MAX - Stabilisation Time":string, "Get Average Delta Tmag (LSIdelta_FISFdelta_LSItmag_FISFtmag_IIRtmag)":string, "Get Average Delta Tmag FISF":string, "MAX - DDM Parameter - Voltage":string, "MAX - DDM Parameter - Current":string, "MAX - DDM Parameter - Power":string, "MAX - DDM Parameter - Measured Power":string, "MAX - DDM Parameter - Speed":string, "MAX - DDM Parameter - Pressure":string, "MAX - Tester Parameter - Voltage":string, "MAX - Tester Parameter - Current":string, "MAX - Tester Parameter - Power":string, "MAX - Tester Parameter - Ambient Pressure":string, "MAX - Tester Parameter - Ambient Temperature":string, "MAX - Tester Parameter - Ambient Humidity":string, "MAX - Calculated Parameter - DDM Pressure Corrected":string, "MAX - Calculated Parameter - DDM Real Power":string, "MAX - Calculated Parameter - Delta V":string, "MAX - Calculated Parameter - Flowrate":string, "MAX - Calculated Parameter - Airwatt":string, "MAX_FISF_Check_Average_Delta_Tmag":string, "MAX - FISF - BEMF Finetune Result":string, "MAX tune - Delta P1":string, "MAX tune - Calculated Parameter - Airwatt":string, "Calculate Delta Airwatts - MAX finetune - Delta P2":string, "MAX finetune - DDM Parameter - Voltage":string, "MAX finetune - DDM Parameter - Current":string, "MAX finetune - DDM Parameter - Power":string, "MAX finetune - DDM Parameter - Measured Power":string, "MAX finetune - DDM Parameter - Speed":string, "MAX finetune - DDM Parameter - Pressure":string, "MAX finetune - Tester Parameter - Voltage":string, "MAX finetune - Tester Parameter - Current":string, "MAX finetune - Tester Parameter - Power":string, "MAX finetune - Tester Parameter - Ambient Pressure":string, "MAX finetune - Tester Parameter - Ambient Temperature":string, "MAX finetune - Tester Parameter - Ambient Humidity":string, "MAX finetune - Calculated Parameter - DDM Pressure Corrected":string, "MAX finetune - Calculated Parameter - DDM Real Power":string, "MAX finetune - Calculated Parameter - Delta V":string, "MAX finetune - Calculated Parameter - Flowrate":string, "MAX finetune - Calculated Parameter - Airwatt":string, "Check Derate Result":string, "Delta Tmag FISF":string, "Get Hot BEMF Result":string, "Calculate delta Pressure":string, "Finalise Calibration":string, "Calculate & Check Delta BEMF":string, "Delta P Airwatts Value":string}, "LL":cluster{"DDM Ambient Temp":string, "Restriction Plate Diameter":string, "LL - DDM Parameter - Voltage":string, "LL - DDM Parameter - Current":string, "LL - DDM Parameter - Power":string, "LL - DDM Parameter - Measured Power":string, "LL - DDM Parameter - Speed":string, "LL - DDM Parameter - Pressure":string, "LL - Tester Parameter - Voltage":string, "LL - Tester Parameter - Current":string, "LL - Tester Parameter - Power":string, "LL - DDM Real Power":string, "LL - Calibrate Task Detect LL":string}, "HL":cluster{"HL - DDM Parameter - Voltage":string, "HL - DDM Parameter - Current":string, "HL - DDM Parameter - Power":string, "HL - DDM Parameter - Measured Power":string, "HL - DDM Parameter - Speed":string, "HL - DDM Parameter - Pressure":string, "HL - Tester Parameter - Voltage":string, "HL - Tester Parameter - Current":string, "HL - Tester Parameter - Power":string, "HL - DDM Real Power":string, "HL - Calibrate Task Detect HL":string}, "LH":cluster{"Restriction Plate Diameter":string, "LH - DDM Parameter - Voltage":string, "LH - DDM Parameter - Current":string, "LH - DDM Parameter - Power":string, "LH - DDM Parameter - Measured Power":string, "LH - DDM Parameter - Speed":string, "LH - DDM Parameter - Pressure":string, "LH - Tester Parameter - Voltage":string, "LH - Tester Parameter - Current":string, "LH - Tester Parameter - Power":string, "LH - DDM Real Power":string, "LH - Calibrate Task Detect LH":string}, "HH":cluster{"HH - DDM Parameter - Voltage":string, "HH - DDM Parameter - Current":string, "HH - DDM Parameter - Power":string, "HH - DDM Parameter - Measured Power":string, "HH - DDM Parameter - Speed":string, "HH - DDM Parameter - Pressure":string, "HH - Tester Parameter - Voltage":string, "HH - Tester Parameter - Current":string, "HH - Tester Parameter - Power":string, "HH - DDM Real Power":string, "HH - Calibrate Task Detect HH":string}, "Inlet Blockage Calibration":cluster{"Inlet Blockage Calibration - DDM Parameter - Voltage":string, "Inlet Blockage Calibration - DDM Parameter - Current":string, "Inlet Blockage Calibration - DDM Parameter - Power":string, "Inlet Blockage Calibration - DDM Parameter - Measured Power":string, "Inlet Blockage Calibration - DDM Parameter - Speed":string, "Inlet Blockage Calibration - DDM Parameter - Pressure":string, "Inlet Blockage Calibration - Tester Parameter - Voltage":string, "Inlet Blockage Calibration - Tester Parameter - Current":string, "Inlet Blockage Calibration - Tester Parameter - Power":string, "Inlet Blockage Calibration - DDM Real Power":string, "Calibration Inlet Blockage_E":string, "Finalise Calibration":string, "Get Task Detect LL":string, "Get Task Detect HL":string, "Get Task Detect LH":string, "Get Task Detect HH":string, "Calibration Inlet Blockage":string, "Calibration eol cold bemf temp":string}, "GOOD":cluster{"GOOD UNIT - Clear EEPROM Error Log":string, "GOOD UNIT - Write Product Timestamp - Mode":string, "GOOD UNIT - Write Product Timestamp - Timestamp":string, "GOOD UNIT - Write Product Timestamp - Rig ID":string, "GOOD UNIT - Write Product Timestamp - Passmark ID":string, "GOOD UNIT - Write Product Timestamp - Passmark Rev":string, "GOOD UNIT - Set Device Mode to PROD":string, "GOOD UNIT - Backup PCBA Calibration EEPROM Response":string, "GOOD UNIT - Check Security Bit":string, "GOOD UNIT - Set Calibration Lock":string, "GOOD UNIT - Get_Calibration_Lock":string, "GOOD UNIT - Disconnect UUT":string}, "NG":cluster{"NG UNIT - Read NVM Error":string, "NG UNIT - Set Device Mode to FCT":string, "NG UNIT - Backup PCBA Calibration EEPROM Response - CAL":string, "NG UNIT - Backup PCBA Calibration EEPROM Response - ERROR":string, "NG UNIT - Backup PCBA Calibration EEPROM Response - USAGE":string, "NG UNIT - Disconnect UUT":string}, "SN":string, "Table":string[][], "Count":cluster{"Total":i32, "OK":i32, "NG":i32, "Yield":dbl}, "Start Time":timestamp, "daemon reference":refnum<k5>, "CT":dbl, "Config":string[][], "OK/NG":bool, "Station ID":string, "MES DDM SN":string, "MES PCBA SN":string, "Retest":string, "Lux":string, "Initialisation_Status":cluster{"LMT - Connect UUT (con COM)":string, "LMT - Software Version (rrel)":string, "LMT - Write SKU file (wskuc)":string, "LMT - SKU file name":string, "Connect UUT DDM":string, "Read DDM EOL Timestamp - Mode":string, "Read DDM EOL Timestamp - Timestamp":string, "Read DDM EOL Timestamp - Rig ID":string, "Read DDM EOL Timestamp - Passmark ID":string, "Read DDM EOL Timestamp - Passmark Rev":string, "Software Version before flashing":string, "Read Hardware Serial":string, "UUT DDM SN":string, "Compare DDM SN with MES SN":string, "Backup PCBA Calibration EEPROM Response - CAL":string, "Flash Firmware Version":string, "Check SW Version":string, "Read DDM SW Version after flashing":string, "Set SKU Config":string, "Ready Status":string, "Set Device Mode to EOL":string, "DDM Parameter - Voltage":string, "DDM Parameter - Current":string, "DDM Parameter - Power":string, "DDM Parameter - Speed":string, "DDM Parameter - Pressure":string, "Tester Parameter - Voltage":string, "Tester Parameter - Current":string, "Tester Parameter - Power":string, "Tester Parameter - Ambient Pressure":string, "Tester Parameter - Ambient Temperature":string, "Calculated Parameter - DDM Pressure Corrected":string, "Calculated Parameter - DDM Real Power":string, "Calculated Parameter - Delta V":string}, "BEMF_Calibration_Status":cluster{"Calibration Result - eol_cold_bemf_temp":string, "DDM Ambient Temp":string, "Restriction Plate Diameter":string, "Calibration Result - eol_bemf_mp_cold_coef_a":string, "Calibration Result - eol_bemf_mp_cold_coef_b":string, "Calibration Result - eol_bemf_mp_cold_coef_c":string, "Calibration Result - eol_bemf_lsi_cold_ref_coeffs":string, "Get - Calibration Result - eol_bemf_lsi_speed":string, "Get - Calibration Result - eol_bemf_lsi_integral_0":string, "Calibration Result - eol_bemf_lsi_integral_1":string, "Get - Calibration Result - eol_bemf_lsi_integral_2":string, "Get - Calibration Result - eol_cold_bemf":string, "Get - Calibration Result - eol_cold_bemf_fisf":string, "Finalise Calibration":string, "Compare -Calibration Result - eol_cold_bemf":string, "Compare -Calibration Result - eol_cold_bemf_fisf":string}, "ECO_Status":cluster{"Reset Power Tune":string, "Reset BEMF FISF Calibration":string, "Restriction Plate Diameter":string, "ECO - Stabilisation Time":string, "ECO - DDM Parameter - Voltage":string, "ECO - DDM Parameter - Current":string, "ECO - DDM Parameter - Power":string, "ECO - DDM Parameter - Measured Power":string, "ECO - DDM Parameter - Speed":string, "ECO - DDM Parameter - Pressure":string, "ECO - Tester Parameter - Voltage":string, "ECO - Tester Parameter - Current":string, "ECO - Tester Parameter - Power":string, "ECO - Tester Parameter - Ambient Pressure":string, "ECO - Tester Parameter - Ambient Temperature":string, "ECO - Tester Parameter - Ambient Humidity":string, "ECO - Calculated Parameter - DDM Pressure Corrected":string, "ECO - Calculated Parameter - DDM Real Power":string, "ECO - Calculated Parameter - Delta V":string, "ECO - Calculated Parameter - Flowrate":string, "ECO - Calculated Parameter - Airwatt":string, "ECO - Formula":string, "PT ECO - Power Tune Mode Status":string}, "BOOST_Status":cluster{"Restriction Plate Diameter":string, "BOOST - Stabilisation Time":string, "BOOST - DDM Parameter - Voltage":string, "BOOST - DDM Parameter - Current":string, "BOOST - DDM Parameter - Power":string, "BOOST - DDM Parameter - Measured Power":string, "BOOST - DDM Parameter - Speed":string, "BOOST - DDM Parameter - Pressure":string, "BOOST - Tester Parameter - Voltage":string, "BOOST - Tester Parameter - Current":string, "BOOST - Tester Parameter - Power":string, "BOOST - Tester Parameter - Ambient Pressure":string, "BOOST - Tester Parameter - Ambient Temperature":string, "BOOST - Tester Parameter - Ambient Humidity":string, "BOOST - Calculated Parameter - DDM Pressure Corrected":string, "BOOST - Calculated Parameter - DDM Real Power":string, "BOOST - Calculated Parameter - Delta V":string, "BOOST - Calculated Parameter - Flowrate":string, "BOOST - Calculated Parameter - Airwatt":string, "BOOST - Get AM Presence":string, "Air Muscle Turn Off Status":string, "BOOST - Air Muscle Calculated Parameter - Airwatt B":string, "BOOST - Air Muscle Calculate Airwatt Delta":string, "PT BOOST - Power Tune Mode Status":string, "Finalise Calibration":string, "ECO - Get AW Calibration value":string, "BOOST - Get AW Calibration value":string}, "MAX_Status":cluster{"Restriction Plate Diameter":string, "MAX - Stabilisation Time":string, "Get Average Delta Tmag (LSIdelta_FISFdelta_LSItmag_FISFtmag_IIRtmag)":string, "Get Average Delta Tmag FISF":string, "MAX - DDM Parameter - Voltage":string, "MAX - DDM Parameter - Current":string, "MAX - DDM Parameter - Power":string, "MAX - DDM Parameter - Measured Power":string, "MAX - DDM Parameter - Speed":string, "MAX - DDM Parameter - Pressure":string, "MAX - Tester Parameter - Voltage":string, "MAX - Tester Parameter - Current":string, "MAX - Tester Parameter - Power":string, "MAX - Tester Parameter - Ambient Pressure":string, "MAX - Tester Parameter - Ambient Temperature":string, "MAX - Tester Parameter - Ambient Humidity":string, "MAX - Calculated Parameter - DDM Pressure Corrected":string, "MAX - Calculated Parameter - DDM Real Power":string, "MAX - Calculated Parameter - Delta V":string, "MAX - Calculated Parameter - Flowrate":string, "MAX - Calculated Parameter - Airwatt":string, "MAX_FISF_Check_Average_Delta_Tmag":string, "MAX - FISF - BEMF Finetune Result":string, "MAX tune - Delta P1":string, "MAX tune - Calculated Parameter - Airwatt":string, "Calculate Delta Airwatts - MAX finetune - Delta P2":string, "MAX finetune - DDM Parameter - Voltage":string, "MAX finetune - DDM Parameter - Current":string, "MAX finetune - DDM Parameter - Power":string, "MAX finetune - DDM Parameter - Measured Power":string, "MAX finetune - DDM Parameter - Speed":string, "MAX finetune - DDM Parameter - Pressure":string, "MAX finetune - Tester Parameter - Voltage":string, "MAX finetune - Tester Parameter - Current":string, "MAX finetune - Tester Parameter - Power":string, "MAX finetune - Tester Parameter - Ambient Pressure":string, "MAX finetune - Tester Parameter - Ambient Temperature":string, "MAX finetune - Tester Parameter - Ambient Humidity":string, "MAX finetune - Calculated Parameter - DDM Pressure Corrected":string, "MAX finetune - Calculated Parameter - DDM Real Power":string, "MAX finetune - Calculated Parameter - Delta V":string, "MAX finetune - Calculated Parameter - Flowrate":string, "MAX finetune - Calculated Parameter - Airwatt":string, "Check Derate Result":string, "Delta Tmag FISF":string, "Get Hot BEMF Result":string, "Calculate delta Pressure":string, "Finalise Calibration":string, "Calculate & Check Delta BEMF":string, "Delta P Airwatts Value":string}, "LL_Status":cluster{"DDM Ambient Temp":string, "Restriction Plate Diameter":string, "LL - DDM Parameter - Voltage":string, "LL - DDM Parameter - Current":string, "LL - DDM Parameter - Power":string, "LL - DDM Parameter - Measured Power":string, "LL - DDM Parameter - Speed":string, "LL - DDM Parameter - Pressure":string, "LL - Tester Parameter - Voltage":string, "LL - Tester Parameter - Current":string, "LL - Tester Parameter - Power":string, "LL - DDM Real Power":string, "LL - Calibrate Task Detect LL":string}, "HL_Status":cluster{"HL - DDM Parameter - Voltage":string, "HL - DDM Parameter - Current":string, "HL - DDM Parameter - Power":string, "HL - DDM Parameter - Measured Power":string, "HL - DDM Parameter - Speed":string, "HL - DDM Parameter - Pressure":string, "HL - Tester Parameter - Voltage":string, "HL - Tester Parameter - Current":string, "HL - Tester Parameter - Power":string, "HL - DDM Real Power":string, "HL - Calibrate Task Detect HL":string}, "LH_Status":cluster{"Restriction Plate Diameter":string, "LH - DDM Parameter - Voltage":string, "LH - DDM Parameter - Current":string, "LH - DDM Parameter - Power":string, "LH - DDM Parameter - Measured Power":string, "LH - DDM Parameter - Speed":string, "LH - DDM Parameter - Pressure":string, "LH - Tester Parameter - Voltage":string, "LH - Tester Parameter - Current":string, "LH - Tester Parameter - Power":string, "LH - DDM Real Power":string, "LH - Calibrate Task Detect LH":string}, "HH_Status":cluster{"HH - DDM Parameter - Voltage":string, "HH - DDM Parameter - Current":string, "HH - DDM Parameter - Power":string, "HH - DDM Parameter - Measured Power":string, "HH - DDM Parameter - Speed":string, "HH - DDM Parameter - Pressure":string, "HH - Tester Parameter - Voltage":string, "HH - Tester Parameter - Current":string, "HH - Tester Parameter - Power":string, "HH - DDM Real Power":string, "HH - Calibrate Task Detect HH":string}, "Inlet Blockage Calibration_Status":cluster{"Inlet Blockage Calibration - DDM Parameter - Voltage":string, "Inlet Blockage Calibration - DDM Parameter - Current":string, "Inlet Blockage Calibration - DDM Parameter - Power":string, "Inlet Blockage Calibration - DDM Parameter - Measured Power":string, "Inlet Blockage Calibration - DDM Parameter - Speed":string, "Inlet Blockage Calibration - DDM Parameter - Pressure":string, "Inlet Blockage Calibration - Tester Parameter - Voltage":string, "Inlet Blockage Calibration - Tester Parameter - Current":string, "Inlet Blockage Calibration - Tester Parameter - Power":string, "Inlet Blockage Calibration - DDM Real Power":string, "Calibration Inlet Blockage_E":string, "Finalise Calibration":string, "Get Task Detect LL":string, "Get Task Detect HL":string, "Get Task Detect LH":string, "Get Task Detect HH":string, "Calibration Inlet Blockage":string, "Calibration eol cold bemf temp":string}, "GOOD_Status":cluster{"GOOD UNIT - Clear EEPROM Error Log":string, "GOOD UNIT - Write Product Timestamp - Mode":string, "GOOD UNIT - Write Product Timestamp - Timestamp":string, "GOOD UNIT - Write Product Timestamp - Rig ID":string, "GOOD UNIT - Write Product Timestamp - Passmark ID":string, "GOOD UNIT - Write Product Timestamp - Passmark Rev":string, "GOOD UNIT - Set Device Mode to PROD":string, "GOOD UNIT - Backup PCBA Calibration EEPROM Response":string, "GOOD UNIT - Check Security Bit":string, "GOOD UNIT - Set Calibration Lock":string, "GOOD UNIT - Get_Calibration_Lock":string, "GOOD UNIT - Disconnect UUT":string}, "NG_Status":cluster{"NG UNIT - Read NVM Error":string, "NG UNIT - Set Device Mode to FCT":string, "NG UNIT - Backup PCBA Calibration EEPROM Response - CAL":string, "NG UNIT - Backup PCBA Calibration EEPROM Response - ERROR":string, "NG UNIT - Backup PCBA Calibration EEPROM Response - USAGE":string, "NG UNIT - Disconnect UUT":string}, "SKU":string, "Plate_Diameter":string, "Alarm":string}
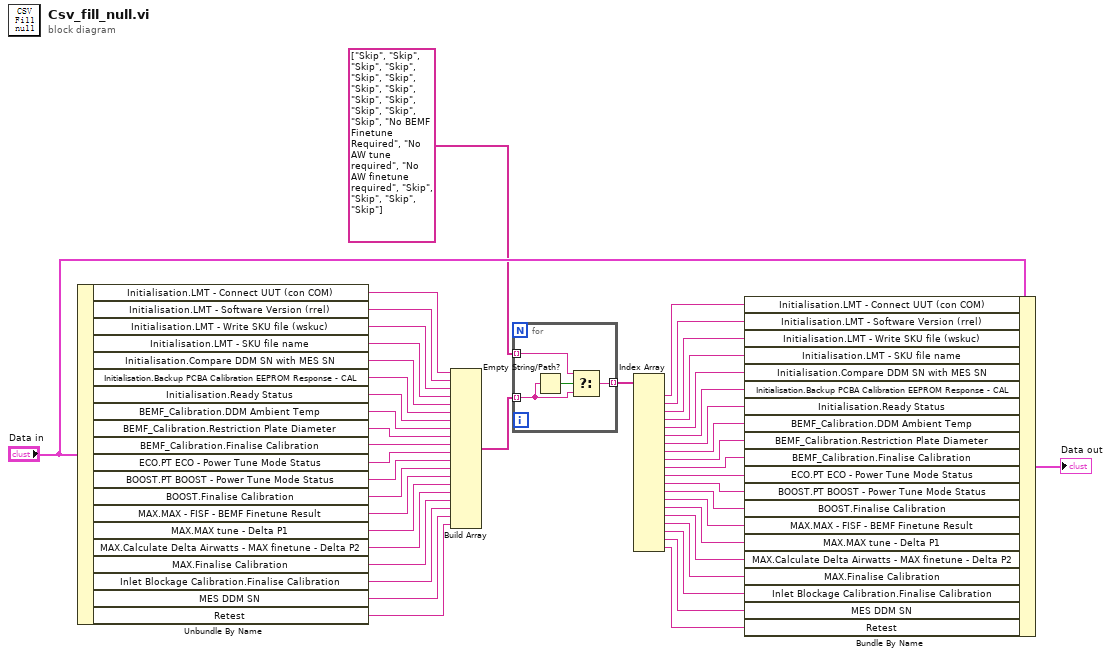
[diagram p0: block diagram]
diagram:
  n1 = Unbundle By Name("Data in") -> ("Initialisation.LMT - Connect UUT (con COM)"=w23:string, "Initialisation.LMT - Software Version (rrel)"=w22:string, "Initialisation.LMT - Write SKU file (wskuc)"=w21:string, "Initialisation.LMT - SKU file name"=w20:string, "Initialisation.Compare DDM SN with MES SN"=w19:string, "Initialisation.Backup PCBA Calibration EEPROM Response - CAL"=w18:string, "Initialisation.Ready Status"=w17:string, "BEMF_Calibration.DDM Ambient Temp"=w16:string, "BEMF_Calibration.Restriction Plate Diameter"=w15:string, "BEMF_Calibration.Finalise Calibration"=w14:string, "ECO.PT ECO - Power Tune Mode Status"=w13:string, "BOOST.PT BOOST - Power Tune Mode Status"=w12:string, "BOOST.Finalise Calibration"=w11:string, "MAX.MAX - FISF - BEMF Finetune Result"=w10:string, "MAX.MAX tune - Delta P1"=w9:string, "MAX.Calculate Delta Airwatts - MAX finetune - Delta P2"=w8:string, "MAX.Finalise Calibration"=w7:string, "Inlet Blockage Calibration.Finalise Calibration"=w6:string, "MES DDM SN"=w5:string, "Retest"=w4:string)
  n2 = Build Array(w23, w22, w21, w20, w19, w18, w17, w16, w15, w14, w13, w12, w11, w10, w9, w8, w7, w6, w5, w4) -> (w3:string[])
  n3 = for {
    tunnel: w3 -> [w47] mode=indexing
    tunnel: string[] ["Skip", "Skip", "Skip", "Skip", "Skip", "Skip", "Skip", "Skip", "Skip", "Skip", "Skip", "Skip", "Skip", "No BEMF Finetune Required", "No AW tune required", "No AW finetune required", "Skip", "Skip", "Skip", "Skip"] ("初始化的数组") -> [w48] mode=indexing
    tunnel: [w46] -> w1 mode=indexing
    n4 = Empty String/Path?(string/path=w47) -> (empty?=w49:bool)
    n5 = Select(t=w48, s=w49, f=w47) -> (s? t:f=w46:string)
  }
  n6 = Index Array(array=w1) -> (element #1=w44:string, element #2=w43:string, element #3=w42:string, element #4=w41:string, element #5=w40:string, element #6=w39:string, element #7=w38:string, element #8=w37:string, element #9=w36:string, element #10=w35:string, element #11=w34:string, element #12=w33:string, element #13=w32:string, element #14=w31:string, element #15=w30:string, element #16=w29:string, element #17=w28:string, element #18=w27:string, element #19=w26:string, element #20=w25:string)  [unwired: 20 in]
  n7 = Bundle By Name(cluster="Data in", "Initialisation.LMT - Connect UUT (con COM)"=w44, "Initialisation.LMT - Software Version (rrel)"=w43, "Initialisation.LMT - Write SKU file (wskuc)"=w42, "Initialisation.LMT - SKU file name"=w41, "Initialisation.Compare DDM SN with MES SN"=w40, "Initialisation.Backup PCBA Calibration EEPROM Response - CAL"=w39, "Initialisation.Ready Status"=w38, "BEMF_Calibration.DDM Ambient Temp"=w37, "BEMF_Calibration.Restriction Plate Diameter"=w36, "BEMF_Calibration.Finalise Calibration"=w35, "ECO.PT ECO - Power Tune Mode Status"=w34, "BOOST.PT BOOST - Power Tune Mode Status"=w33, "BOOST.Finalise Calibration"=w32, "MAX.MAX - FISF - BEMF Finetune Result"=w31, "MAX.MAX tune - Delta P1"=w30, "MAX.Calculate Delta Airwatts - MAX finetune - Delta P2"=w29, "MAX.Finalise Calibration"=w28, "Inlet Blockage Calibration.Finalise Calibration"=w27, "MES DDM SN"=w26, "Retest"=w25) -> (→"Data out":T1)
